vi "LogData.vi"(6 "Run Ratios":T2 {"LEC13/12" format="%_4e"; "DTfrac" format="%#_3g"; "DT" format="%#_3g"; "CountErr" format="%#_3g"; "d13C" format="%_4g"; "C13/12" format="%_4e"; "C14/12" format="%_4e"; "C14/13" format="%_3e"; "C12Cor" format="%_3e"; "C13" format="%_3e"; "C13H/L" format="%#_3g"}, 8 "error in (no error)":errorcluster, 9 "Run Summary":T3 {"C12LE" format="%_3e"; "C13LE" format="%_3e"; "C1312" format="%_3e"; "C12" format="%_3e"; "C13L" format="%_3e"; "C13H" format="%_3e"}, 10 "Sample Data":T1, 11 "Log File Path":path) -> (0 "error out":errorcluster, 1 "Result string":string)   [LabVIEW 2013]
uses:
  SummaryData.ctl
  RunRatios.ctl
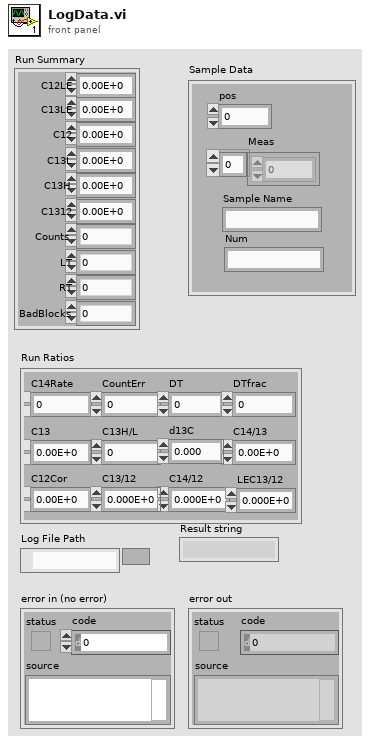
[diagram p1: front panel]
types:
  T1 = cluster{"pos":i32, "Meas":i32[], "Sample Name":string, "Num":string}
  T2 = typedef "RunRatios.ctl" = cluster{"C14Rate":dbl, "CountErr":dbl, "DT":dbl, "DTfrac":dbl, "C13":dbl, "C13H/L":dbl, "d13C":dbl, "C14/13":dbl, "C12Cor":dbl, "C13/12":dbl, "C14/12":dbl, "LEC13/12":dbl}
  T3 = typedef "SummaryData.ctl" = cluster{"C12LE":dbl, "C13LE":dbl, "C12":dbl, "C13L":dbl, "C13H":dbl, "C1312":dbl, "Counts":u32, "LT":dbl, "RT":dbl, "BadBlocks":u8}
  T4 = enum16{"open", "replace", "create", "open or create", "replace or create", "replace or create with confirmation"}
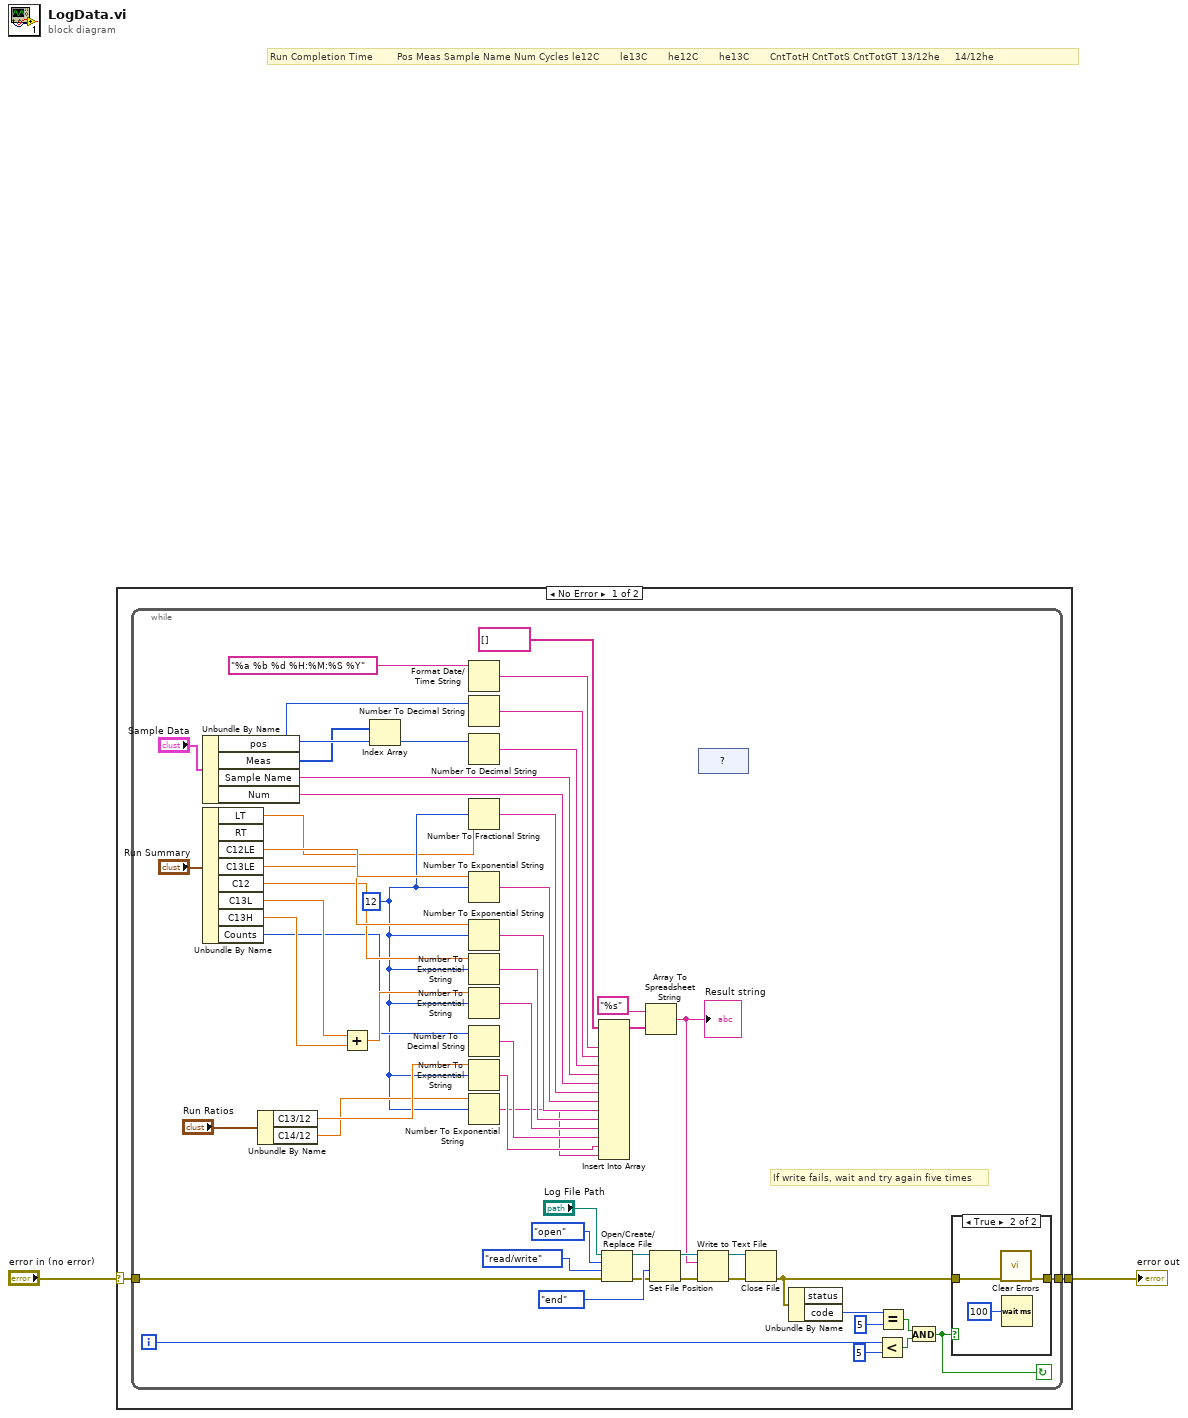
[diagram p0: block diagram]
diagram:
  # "Run Completion Time       \tPos\tMeas\tSample Name\tNum\tCycles\tle12C      \tle13C      \the12C      \the13C      \tCntTotH\tCntTotS\tCntTotGT\t13/12he    \t14/12he"
  n1 = case shown="No Error" "error in (no error)" {
    selector: "error in (no error)" -> [w4 w64]
    tunnel: [w3 w64] -> w1
    frame No Error {
      n2 = while {
        tunnel: w4 -> [w25]
        tunnel: [w10] -> w3
        i -> [w15]
        stop <- w12 continue-if-true
        w19 = i16 12 ("width (-)")
        # "If write fails, wait and try again five times"
        n3 = Unbundle By Name("Sample Data") -> ("pos"=w22:i32, "Meas"=w21:i32[], "Sample Name"=w20:string, "Num"=w9:string)
        n4 = Unbundle By Name("Run Summary") -> ("LT"=w8:dbl, "C12LE"=w38:dbl, "C13LE"=w37:dbl, "C12"=w36:dbl, "C13L"=w35:dbl, "C13H"=w34:dbl, "Counts"=w32:u32)  [unwired: 1 out]
        n5 = Unbundle By Name("Run Ratios") -> ("C13/12"=w30:dbl, "C14/12"=w29:dbl)
        n6 = Add(x=w35, y=w34) -> (x+y=w33:dbl)
        n7 = Index Array(array=w21, index=w22) -> (element=w24:i32)
        n8 = Format Date/Time String(time format string (%c)="%a %b %d %H:%M:%S %Y") -> (date/time string=w58:string)  [unwired: 2 out]
        n9 = Number To Decimal String(number=w22) -> (decimal integer string=w48:string)  [unwired: 1 out]
        n10 = Number To Decimal String(number=w24) -> (decimal integer string=w47:string)  [unwired: 1 out]
        n11 = Number To Fractional String(number=w8, width (-)=w19) -> (F-format string=w46:string)  [unwired: 2 in]
        n12 = Number To Exponential String(number=w38, 3:w19) -> (E-format string=w45:string)  [unwired: 2 in]
        n13 = Number To Exponential String(number=w37, 3:w19) -> (E-format string=w44:string)  [unwired: 2 in]
        n14 = Number To Exponential String(number=w36, 3:w19) -> (E-format string=w43:string)  [unwired: 2 in]
        n15 = Number To Exponential String(number=w33, 3:w19) -> (E-format string=w42:string)  [unwired: 2 in]
        n16 = Number To Decimal String(number=w32) -> (decimal integer string=w7:string)  [unwired: 1 out]
        n17 = Number To Exponential String(number=w30, 3:w19) -> (E-format string=w6:string)  [unwired: 2 in]
        n18 = Number To Exponential String(number=w29, 3:w19) -> (E-format string=w5:string)  [unwired: 2 in]
        n19 = Insert Into Array(array=string[] [], new element #1=w58, new element #2=w48, new element #3=w47, new element #4=w20, new element #5=w9, new element #6=w46, new element #7=w45, new element #8=w44, new element #9=w43, new element #10=w42, new element #11=w7, new element #12=w6, new element #13=w5) -> (w41:string[])  [unwired: 1 in]
        n20 = Open/Create/Replace File(file path (use dialog)="Log File Path", error in=w25, operation (0:open)=T4."open", access (0:read/write)=enum16{"read/write", "read-only", "write-only"}."read/write") -> (refnum out=w51:refnum<file>, error out=w28:errorcluster)  [unwired: 3 out]
        n21 = Array To Spreadsheet String(array=w41, 3:"%s" ("format string")) -> (spreadsheet string=w49:string)  [unwired: 1 out]
        "Result string" <- w49
        n22 = Set File Position(refnum=w51, from (0:start)=enum16{"start", "end", "current"}."end", error in=w28) -> (refnum out=w50:refnum<file>, error out=w27:errorcluster)  [unwired: 1 in]
        n23 = Write to Text File(file (use dialog)=w50, text=w49, error in=w27) -> (refnum out=w56:refnum<file>, error out=w26:errorcluster)  [unwired: 2 out]
        n24 = shared-variable "?"() -> ()  [unwired: 1 in, 2 out]
        n25 = Close File(refnum=w56, error in=w26) -> (error out=w11:errorcluster)  [unwired: 1 out]
        n26 = Unbundle By Name(w11) -> ("code"=w18:i32)  [unwired: 1 out]
        n27 = Less?(x=w15, y=5) -> (x < y?=w16:bool)
        n28 = Equal?(x=w18, y=5) -> (x = y?=w13:bool)
        n29 = And(x=w13, y=w16) -> (x .and. y?=w12:bool)
        n30 = case shown="True" w12 {
          tunnel: [w60 w62] -> w10
          tunnel: w11 -> [w60 w61]
          frame False {
          }
          frame True {
            n31 = call <vilib>:"Clear Errors.vi"("error in (no error)"=w61) -> ("error out"=w62:errorcluster)  [unwired: 6 in]
            n32 = Wait (ms)(milliseconds to wait=u32 100) -> ()  [unwired: 1 out]
          }
        }
      }
    }
    frame Error {
    }
  }
  "error out" <- w1
